vi "Query Trace Data.vi"(8 "error in (no error)":errorcluster, 10 "Trace Number":u8=1, 11 "VNA-ZNB in":refnum<class "VNA-ZNB.lvclass">) -> (0 "error out":errorcluster, 1 "Data":dbl[](array[numeric]), 2 "Frequency":dbl[](array[numeric]), 3 "VNA-ZNB out":refnum<class "VNA-ZNB.lvclass">)   [LabVIEW 2020, in "VNA-ZNB.lvclass"]
doc: "Query the active trace data.\nIt returns both x and y data"
uses:
  VNA-ZNB.lvclass
  C:/Sandbox/RF Bench/Source Code/WiSpry Test Framework/Instruments/Instrument.lvclass
  C:/Sandbox/RF Bench/Source Code/WiSpry Test Framework/Instruments/Vector Network Analyzer/Vector Network Analyzer.lvclass
  Vector Network Analyzer.lvclass/Vector Network Analyzer.ctl
  Instrument.lvclass/Instrument.ctl
  Instrument.lvclass
  Vector Network Analyzer.lvclass
panel:
  out "size(s)":i32
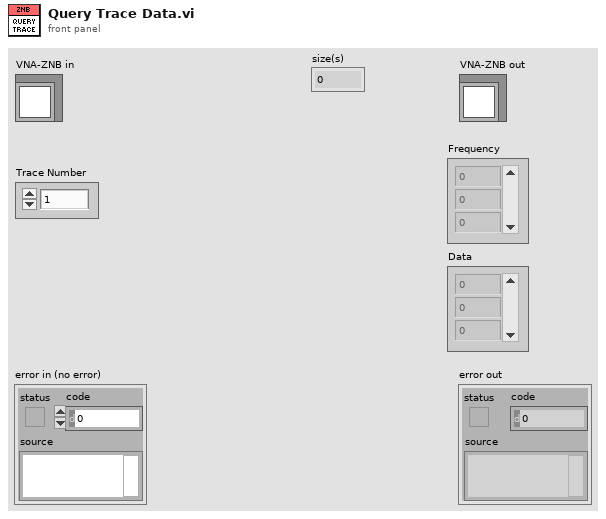
[diagram p1: front panel]
types:
  T1 = enum16{"big-endian, network order", "native, host order", "little-endian"}
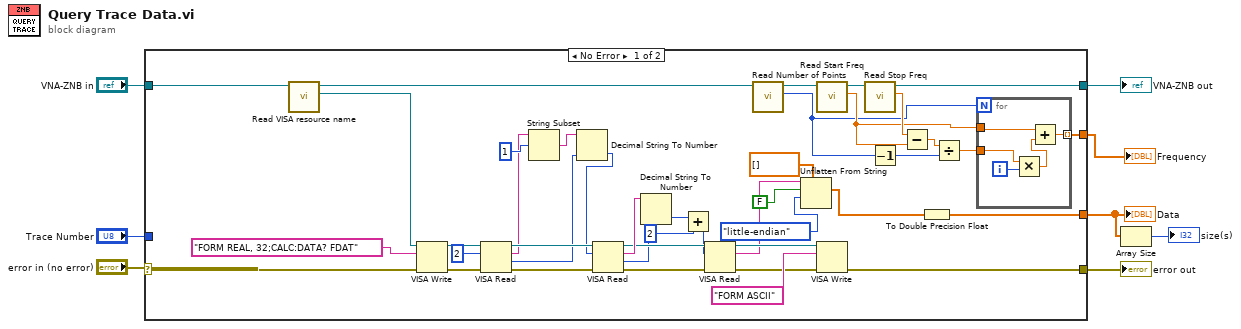
[diagram p0: block diagram]
diagram:
  n1 = case shown="No Error" "error in (no error)" {
    selector: "error in (no error)" -> [w49 w57]
    tunnel: "Trace Number" -> [_ _]
    tunnel: "VNA-ZNB in" -> [w50 w56]
    tunnel: [w30 w57] -> w5
    tunnel: [w37 w56] -> w4
    tunnel: [w32 _] -> w3
    tunnel: [w15 _] -> w1
    frame No Error {
      n2 = call "Read VISA resource name.vi"("Instrument in"=w50) -> ("VISA resource name"=w48:refnum<visa-resource-name>, "Instrument out"=w40:refnum<class "VNA-ZNB.lvclass">)  [unwired: 9 in]
      n3 = VISA Write(VISA resource name=w48, write buffer="FORM REAL, 32;CALC:DATA? FDAT" ("initial string"), error in (no error)=w49) -> (VISA resource name out=w46:refnum<visa-resource-name>, error out=w47:errorcluster)  [unwired: 1 out]
      n4 = VISA Read(VISA resource name=w46, byte count=u32 2, error in (no error)=w47) -> (VISA resource name out=w43:refnum<visa-resource-name>, read buffer=w21:string, return count=w42:u32, error out=w44:errorcluster)
      n5 = String Subset(string=w21, offset (0)=1) -> (substring=w23:string)  [unwired: 1 in]
      n6 = Decimal String To Number(string=w23, default (0L)=w42) -> (number=w13:u32)  [unwired: 1 in, 1 out]
      n7 = VISA Read(VISA resource name=w43, byte count=w13, error in (no error)=w44) -> (VISA resource name out=w28:refnum<visa-resource-name>, read buffer=w29:string, return count=w20:u32, error out=w27:errorcluster)
      n8 = Decimal String To Number(string=w29, default (0L)=w20) -> (number=w24:u32)  [unwired: 1 in, 1 out]
      n9 = Add(x=w24, y=u32 2) -> (x+y=w12:u32)
      n10 = VISA Read(VISA resource name=w28, byte count=w12, error in (no error)=w27) -> (VISA resource name out=w25:refnum<visa-resource-name>, read buffer=w19:string, error out=w26:errorcluster)  [unwired: 1 out]
      n11 = call "Read Number of Points.vi"("Vector Network Analyzer in"=w40) -> ("Number of Points"=w9:i32, "Vector Network Analyzer out"=w39:refnum<class "VNA-ZNB.lvclass">)  [unwired: 9 in]
      n12 = Unflatten From String(type=sgl[] [], binary string=w19, data includes array or string size? (T)=FALSE, byte order (0:big-endian, network order)=T1."little-endian") -> (value=w16:sgl[])  [unwired: 1 in, 2 out]
      n13 = call "Read Start Freq.vi"("Vector Network Analyzer in"=w39) -> ("Start Freq"=w34:dbl, "Vector Network Analyzer out"=w38:refnum<class "VNA-ZNB.lvclass">)  [unwired: 9 in]
      n14 = VISA Write(VISA resource name=w25, write buffer="FORM ASCII", error in (no error)=w26) -> (error out=w30:errorcluster)  [unwired: 2 out]
      n15 = call "Read Stop Freq.vi"("Vector Network Analyzer in"=w38) -> ("Stop Freq"=w36:dbl, "Vector Network Analyzer out"=w37:refnum<class "VNA-ZNB.lvclass">)  [unwired: 9 in]
      n16 = Decrement(x=w9) -> (x-1=w10:i32)
      n17 = Subtract(x=w36, y=w34) -> (x-y=w35:dbl)
      n18 = To Double Precision Float(number=w16) -> (double precision float=w15:dbl[])
      n19 = Divide(x=w35, y=w10) -> (x/y=w33:dbl)
      n20 = for {
        N: w9 -> [_]
        tunnel: w34 -> [w52]
        tunnel: w33 -> [w54]
        tunnel: [w51] -> w32 mode=indexing
        i -> [w55]
        n21 = Multiply(x=w54, y=w55) -> (x*y=w53:dbl)
        n22 = Add(x=w52, y=w53) -> (x+y=w51:dbl)
      }
    }
    frame Error {
    }
  }
  "error out" <- w5
  "VNA-ZNB out" <- w4
  "Data" <- w1
  "Frequency" <- w3
  n23 = Array Size(array=w1) -> (size(s)=→"size(s)":i32)
